vi "Add Resolver.vi"(8 "error in (no error)":errorcluster, 10 "HTTP Server:TemplateVariableResolver.lvclass":refnum<class "TemplateVariableResolver.lvclass">, 11 "BasicTemplater in":refnum<class "BasicTemplater.lvclass">) -> (0 "error out":errorcluster, 3 "BasicTemplater out":refnum<class "BasicTemplater.lvclass">)   [LabVIEW 2020, in "HTTP Server.lvlib" / "BasicTemplater.lvclass"]
uses:
  BasicTemplater.lvclass
  BasicTemplater.lvclass/BasicTemplater.ctl
  TemplateVariableResolver/TemplateVariableResolver.lvclass
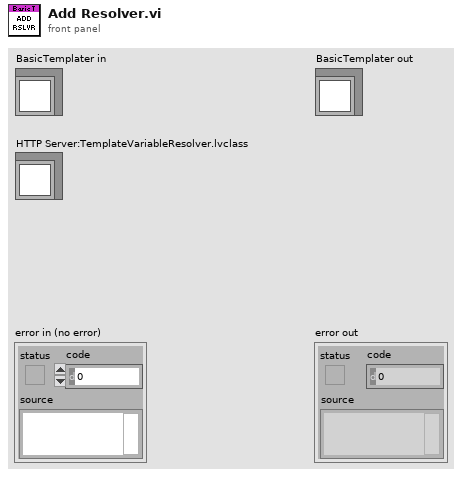
[diagram p1: front panel]
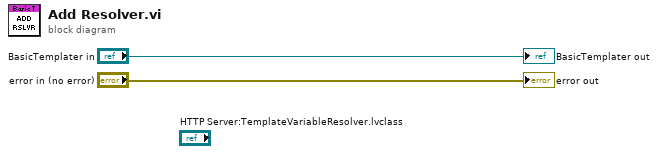
[diagram p0: block diagram]
diagram:
  "error out" <- "error in (no error)"
  "BasicTemplater out" <- "BasicTemplater in"
